vi "ConvertXYgraph.vi"(7 "Buffer Size (1000)":i32=1000, 10 "Last Row":i32, 11 "Raw Data":dbl[][](array[numeric])) -> (3 "Output":cluster{"x":dbl, "y":dbl}[](array[cluster]))   [LabVIEW 2011]
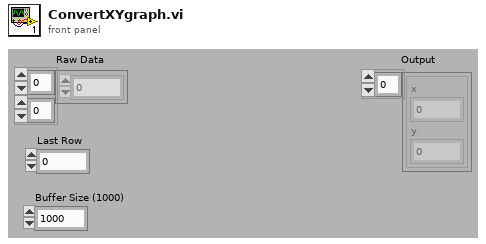
[diagram p1: front panel]
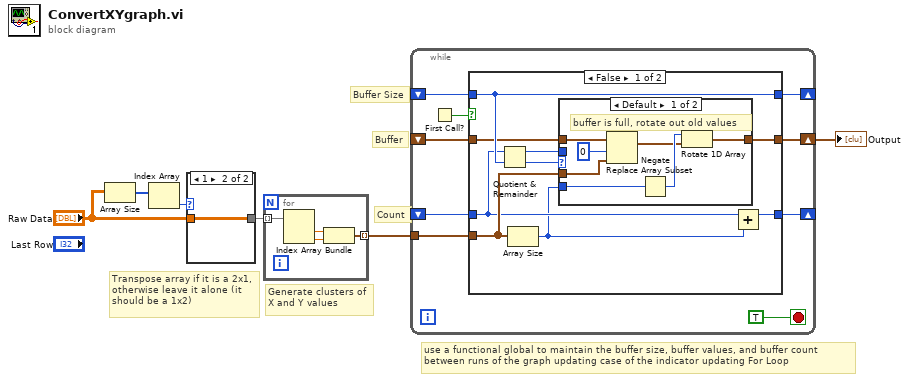
[diagram p0: block diagram]
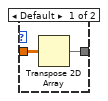
[diagram p2: hidden frame]
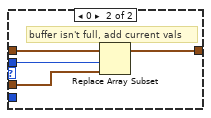
[diagram p3: hidden frame]
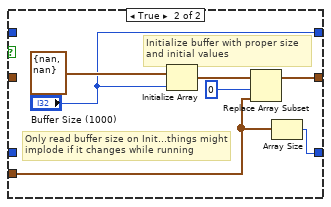
[diagram p4: hidden frame]
diagram:
  # "use a functional global to maintain the buffer size, buffer values, and buffer count\nbetween runs of the graph updating case of the indicator updating For Loop"
  # "Generate clusters of\nX and Y values"
  # "Transpose array if it is a 2x1,\notherwise leave it alone (it\nshould be a 1x2)"
  # "Buffer Size"
  # "Count"
  # "Buffer"
  n1 = Array Size(array="Raw Data") -> (size(s)=w4:i32[])
  n2 = Index Array(array=w4) -> (element=w2:i32)  [unwired: 1 in]
  n3 = case shown="1" w2 {
    tunnel: "Raw Data" -> [w7 w9]
    tunnel: [w8 w9] -> w1
    frame Default {
      n4 = Transpose 2D Array(2D array=w7) -> (transposed array=w8:dbl[][])
    }
    frame 1 {
    }
  }
  n5 = for {
    tunnel: w1 -> [w13] mode=indexing
    tunnel: [w10] -> w5 mode=indexing
    n6 = Index Array(array=w13) -> (element #1=w11:dbl, element #2=w12:dbl)  [unwired: 2 in]
    n7 = Bundle("Numeric"=w11, "Numeric"=w12) -> (w10:cluster{"Numeric":dbl, "Numeric":dbl})  [unwired: 1 out]
  }
  n8 = while {
    shift-right: [w20] -> w6
    shift-left: _ -> [w19]
    tunnel: w5 -> [w18]
    shift-right: [w16] -> _
    shift-left: _ -> [w17]
    shift-right: [w15] -> _
    shift-left: _ -> [w14]
    stop <- TRUE stop-if-true
    n9 = First Call?() -> (First Call?: T/F=w21:bool)
    n10 = case shown="False" w21 {
      tunnel: [w27 w43] -> w20
      tunnel: w19 -> [w28 _]
      tunnel: w18 -> [w26 w44]
      tunnel: w17 -> [w25 _]
      tunnel: [w31 w48] -> w16
      tunnel: [w30 "Buffer Size (1000)"] -> w15
      tunnel: w14 -> [w30 _]
      frame False {
        n11 = Quotient & Remainder(x=w25, y=w30) -> (x-y*floor(x/y)=w24:i32, floor(x/y)=w29:i32)
        n12 = Array Size(array=w26) -> (size(s)=w23:i32)
        n13 = case shown="Default" w29 {
          tunnel: w28 -> [w38 w42]
          tunnel: [w32 w41] -> w27
          tunnel: w26 -> [w37 w40]
          tunnel: w24 -> [_ w39]
          tunnel: w23 -> [w35 _]
          frame Default {
            # "buffer is full, rotate out old values"
            n14 = Replace Array Subset(array=w38, new element=w37, index=0) -> (w33:cluster{"x":dbl, "y":dbl}[])
            n15 = Negate(x=w35) -> (-x=w34:i32)
            n16 = Rotate 1D Array(1:w33, 2:w34) -> (0:w32:cluster{"x":dbl, "y":dbl}[])
          }
          frame 0 {
            # "buffer isn't full, add current vals"
            n17 = Replace Array Subset(array=w42, new element=w40, index=w39) -> (w41:cluster{"x":dbl, "y":dbl}[])
          }
        }
        n18 = Add(x=w25, y=w23) -> (x+y=w31:i32)
      }
      frame True {
        # "Initialize buffer with proper size\nand initial values"
        # "Only read buffer size on Init...things might implode if it changes while running"
        n19 = Initialize Array(cluster{"x":dbl, "y":dbl} {"x"=nan, "y"=nan} ("Cluster"), "Buffer Size (1000)") -> (w47:cluster{"x":dbl, "y":dbl}[])
        n20 = Replace Array Subset(array=w47, new element=w44, index=0) -> (w43:cluster{"x":dbl, "y":dbl}[])
        n21 = Array Size(array=w44) -> (size(s)=w48:i32)
      }
    }
  }
  "Output" <- w6
